vi "Read Multi CDBL.vi"(8 "error in (no error)":errorcluster, 10 "Tag":string[](array[string]), 11 "Var Bus in":refnum<class "Omni_Bus.lvclass">) -> (0 "error out":errorcluster, 2 "Array":cdb[](array[numeric]), 3 "Var Bus out":refnum<class "Omni_Bus.lvclass">)   [LabVIEW 2021, in "Omni_Bus.lvclass"]
uses:
  Omni_Bus.lvclass
  Omni_Bus.lvclass/Omni_Bus.ctl
  <vilib>/TSA/Abstract Data Classes/Abs_Types/Complex Double Float/Abs_Complex Double Float.lvclass
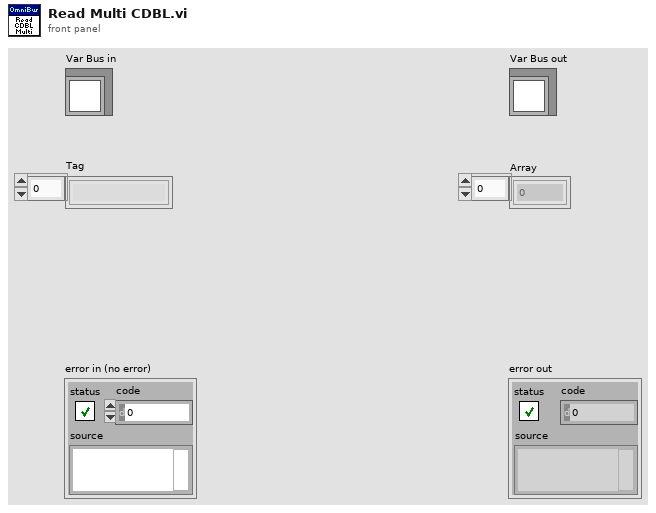
[diagram p1: front panel]
types:
  T1 = typedef "Abs_Complex Double Float.lvclass/Type.ctl" = cdb
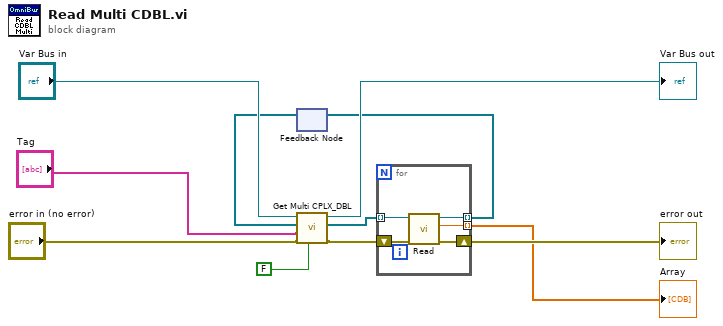
[diagram p0: block diagram]
diagram:
  n1 = feedback #1() -> (w2:refnum<class "Abs_Complex Double Float.lvclass">[])  [unwired: 1 in]
  n2 = call-dynamic "Get Multi CPLX_DBL.vi"("Write?"=FALSE, "error in (no error)"="error in (no error)", "Tag"="Tag", "Value Type"=w2, "Var Bus in"="Var Bus in") -> ("error out"=w4:errorcluster, "Value Out"=w3:refnum<class "Abs_Complex Double Float.lvclass">[], "Var Bus out"=→"Var Bus out":refnum<class "Omni_Bus.lvclass">)  [unwired: 4 in]
  n3 = for {
    tunnel: [w15] -> w6 mode=indexing
    tunnel: [w14] -> w5 mode=indexing
    tunnel: w3 -> [w12] mode=indexing
    shift-right: [w16] -> w10
    shift-left: w4 -> [w13]
    n4 = call-dynamic "Read.vi"("error in (no error)"=w13, "Double Float.lvclass_340760 in"=w12) -> ("error out"=w16:errorcluster, "Value"=w15:T1, "Double Float.lvclass_340760 out"=w14:refnum<class "Abs_Complex Double Float.lvclass">)  [unwired: 7 in]
  }
  "error out" <- w10
  "Array" <- w6
  n5 = feedback-in #1(w5) -> ()
